vi "Write custom timing source_.vi"(8 "error in":errorcluster, 10 "custom timing source?":bool, 11 "DecideProjectFeatures in":refnum<class "UserTBModuleDecideFeatures.lvclass">) -> (0 "error out":errorcluster, 3 "DecideProjectFeatures out":refnum<class "UserTBModuleDecideFeatures.lvclass">)   [LabVIEW 2013, in "UserTBModuleDecideFeatures.lvclass"]
uses:
  UserTBModuleDecideFeatures.lvclass
  UserTBModuleDecideFeatures.lvclass/UserTBModuleDecideFeatures.ctl
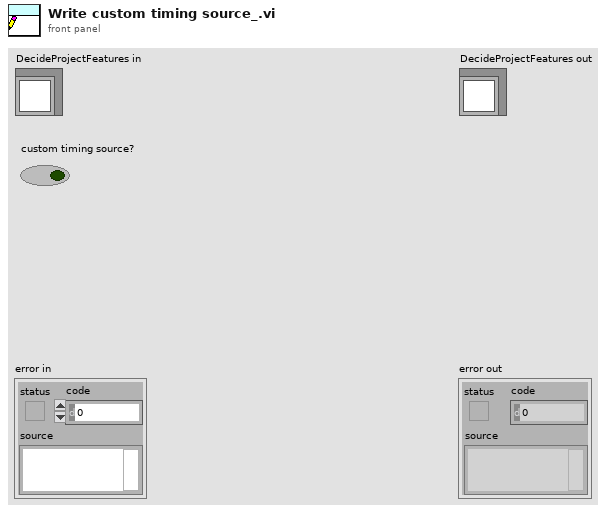
[diagram p1: front panel]
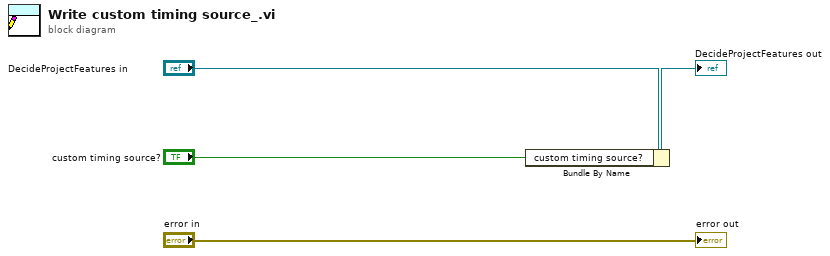
[diagram p0: block diagram]
diagram:
  n1 = Bundle By Name(cluster="DecideProjectFeatures in", "custom timing source?"="custom timing source?") -> (→"DecideProjectFeatures out":refnum<class "UserTBModuleDecideFeatures.lvclass">)
  "error out" <- "error in"
